vi "Teleop.vi"(10 "Match Info":T1={"Autonomous Elapsed Seconds"=0.0, "TeleOp Elapsed Seconds"=0.0, "Disabled Elapsed Seconds"=0.0, "Visited Autonomous"=FALSE, "Visited TeleOp"=FALSE, "Visited Disabled"=FALSE, "Autonomous Settings"={"Autonomous Style"=enum."Independent", "VI Refnum"=refnum}}, 11 "Call Context":T2) -> ()   [LabVIEW 2016]
doc: "This VI is called for each TeleOp packet received from the DS where the robot is not disabled. It is often used to read from the joysticks and update I/O or to update setpoints for timed control loops. It should complete and return within 20 milliseconds or it may miss DS packets."
uses:
  <vilib>/Rock Robotics/WPI/DriverStation/WPI_DriverStationDerivedRobotMode.ctl
  <vilib>/Rock Robotics/WPI/DriverStation/WPI_DriverStationMatch Info.ctl
  <vilib>/Rock Robotics/Network Tables/NT Read Boolean.vi
  <vilib>/Rock Robotics/Network Tables/NT Read Number.vi
  Globals/Constantes.vi
  Globals/InputValues.vi
  Globals/Globals.vi
panel:
  out "output":bool
  out "state":bool
  in  "Dont block":bool
  out "Sample Slider 0":dbl(slide) scale=0.0..5.0
  out "Sample Boolean 1":bool
  out "Sample Boolean 0":bool
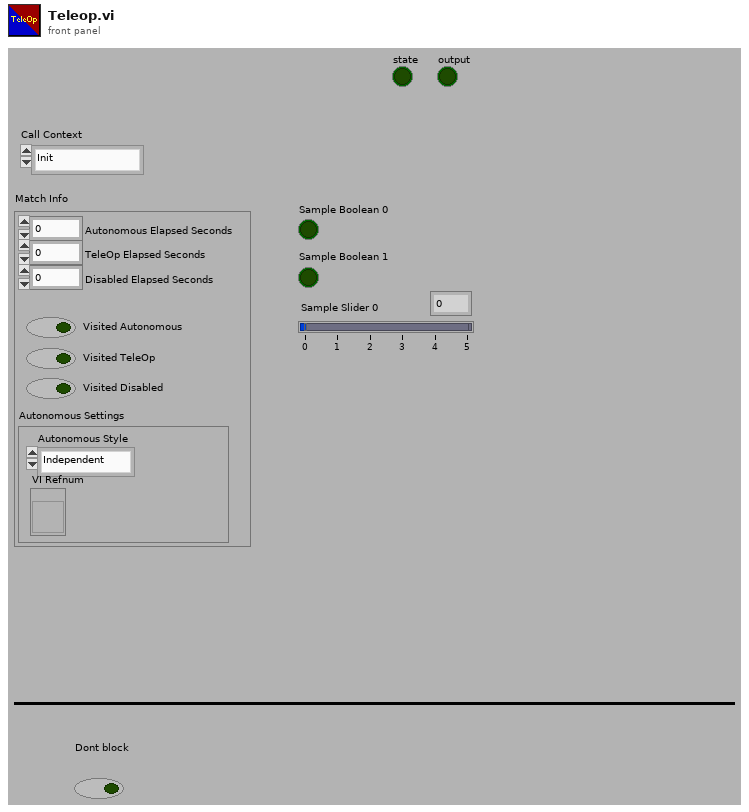
[diagram p1: front panel]
types:
  T1 = typedef "WPI_DriverStationMatch Info.ctl" = cluster{"Autonomous Elapsed Seconds":dbl, "TeleOp Elapsed Seconds":dbl, "Disabled Elapsed Seconds":dbl, "Visited Autonomous":bool, "Visited TeleOp":bool, "Visited Disabled":bool, "Autonomous Settings":cluster{"Autonomous Style":enum16{"Iterative", "Independent"}, "VI Refnum":refnum<vi>}}
  T2 = typedef "WPI_DriverStationDerivedRobotMode.ctl" = enum16{"Init", "Execute", "Stop"}
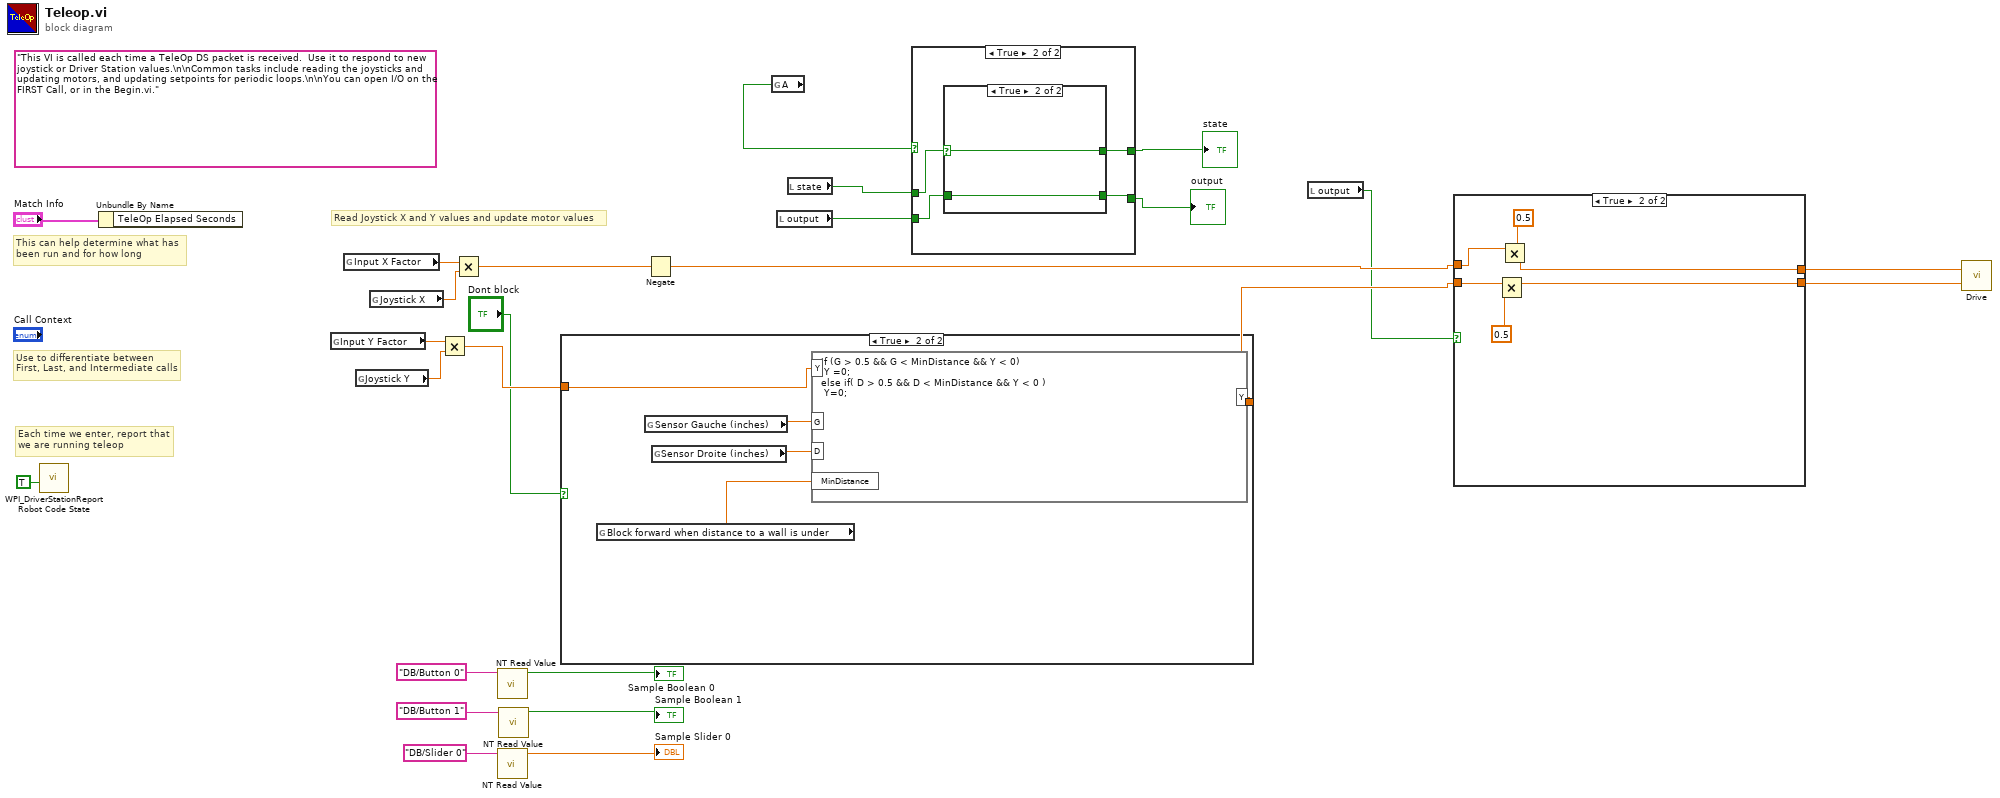
[diagram p0: block diagram]
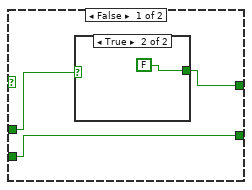
[diagram p2: hidden frame]
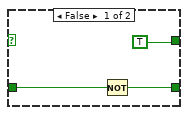
[diagram p4: hidden frame]
diagram:
  (unwired) "This VI is called each time a TeleOp DS packet is received.  Use it to respond to new joystick or Driver Station values.\n\nCommon tasks include reading the joysticks and updating motors, and updating setpoints for periodic loops.\n\nYou can open I/O on the FIRST Call, or in the Begin.vi."
  # "Each time we enter, report that\nwe are running teleop"
  # "Use to differentiate between\nFirst, Last, and Intermediate calls"
  # "This can help determine what has\nbeen run and for how long"
  # "Read Joystick X and Y values and update motor values"
  n1 = call <vilib>:"WPI_DriverStationReport Robot Code State.vi"("TeleOp"=TRUE ("Autonomous")) -> ()  [unwired: 10 in, 1 out]
  n2 = Unbundle By Name("Match Info") -> ()  [unwired: 1 out]
  n3 = global read "Constantes.vi" "Input Y Factor"() -> (w15:dbl)
  n4 = global read "Constantes.vi" "Input X Factor"() -> (w16:dbl)
  n5 = global read "InputValues.vi" "Joystick Y"() -> (w14:dbl)
  n6 = global read "InputValues.vi" "Joystick X"() -> (w13:dbl)
  n7 = Multiply(x=w15, y=w14) -> (x*y=w17:dbl)
  n8 = Multiply(x=w16, y=w13) -> (x*y=w12:dbl)
  n9 = call-poly <vilib>:"NT Read Value.vi"("Name"="DB/Button 0" ("refnum name")) -> ("Boolean"=→"Sample Boolean 0":bool)  [unwired: 9 in, 1 out]
  n10 = call-poly <vilib>:"NT Read Value.vi"("Name"="DB/Slider 0" ("refnum name")) -> ("Numeric"=→"Sample Slider 0":dbl)  [unwired: 9 in, 1 out]
  n11 = call-poly <vilib>:"NT Read Value.vi"("Name"="DB/Button 1" ("refnum name")) -> ("Boolean"=→"Sample Boolean 1":bool)  [unwired: 9 in, 1 out]
  n12 = case shown="True" "Dont block" {
    tunnel: w17 -> [w26 w31]
    tunnel: [w26 w27] -> w9
    frame False {
    }
    frame True {
      n13 = global read "Constantes.vi" "Block forward when distance to a wall is under"() -> (w28:dbl)
      n14 = global read "Globals.vi" "Sensor Gauche (inches)"() -> (w30:dbl)
      n15 = global read "Globals.vi" "Sensor Droite (inches)"() -> (w29:dbl)
      n16 = formula code="if (G > 0.5 && G < MinDistance && Y < 0)\n Y =0;\nelse if( D > 0.5 && D < MinDistance && Y < 0 )\n Y=0;"("G"=w30, "D"=w29, "Y"=w31, "MinDistance"=w28) -> ("Y"=w27:dbl)
    }
  }
  n17 = Negate(x=w12) -> (-x=w10:dbl)
  n18 = global read "InputValues.vi" "A"() -> (w6:bool)
  n19 = local read "output"() -> (w3:bool)
  n20 = local read "state"() -> (w5:bool)
  n21 = case shown="True" w6 {
    tunnel: w5 -> [w34 w40]
    tunnel: [w33 w39] -> w4
    tunnel: w3 -> [w32 w38]
    tunnel: [w32 w37] -> w2
    frame False {
      n22 = case shown="True" w34 {
        selector: w34 -> [w35 _]
        tunnel: [w35 FALSE] -> w33
        frame False {
        }
        frame True {
        }
      }
    }
    frame True {
      n23 = case shown="True" w40 {
        selector: w40 -> [_ w45]
        tunnel: [TRUE w45] -> w39
        tunnel: w38 -> [w42 w44]
        tunnel: [w41 w44] -> w37
        frame False {
          n24 = Not(x=w42) -> (.not. x?=w41:bool)
        }
        frame True {
        }
      }
    }
  }
  "state" <- w4
  "output" <- w2
  n25 = local read "output"() -> (w1:bool)
  n26 = case shown="True" w1 {
    tunnel: w10 -> [w47 w53]
    tunnel: w9 -> [w46 w52]
    tunnel: [w47 w51] -> w8
    tunnel: [w46 w49] -> w7
    frame False {
    }
    frame True {
      n27 = Multiply(x=w52, y=0.5) -> (x*y=w49:dbl)
      n28 = Multiply(x=w53, y=0.5) -> (x*y=w51:dbl)
    }
  }
  n29 = call "Drive.vi"("Y (Forward)"=w7, "X (Rotation)"=w8) -> ()  [unwired: 1 in]
